vi "close.vi"(8 "error in (no error)":errorcluster, 11 "Keysight 33511B in":refnum<class "Keysight 33511B.lvclass">) -> (0 "error out":errorcluster)   [LabVIEW 2020, in "Keysight 33511B.lvclass"]
uses:
  Keysight 33511B.lvclass
  Keysight 33511B.lvclass/Keysight 33511B.ctl
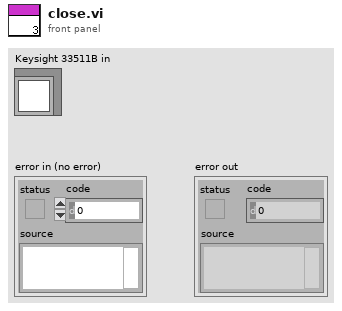
[diagram p1: front panel]
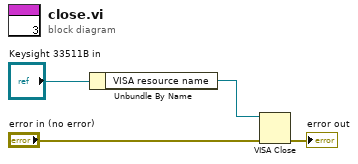
[diagram p0: block diagram]
diagram:
  n1 = Unbundle By Name("Keysight 33511B in") -> ("VISA resource name"=w3:refnum<visa-resource-name>)
  n2 = VISA Close(VISA resource name=w3, error in (no error)="error in (no error)") -> (error out=→"error out":errorcluster)
